vi "Parse Object Content.vi"(8 "error in (no error)":errorcluster, 11 "Response body":string) -> (0 "error out":errorcluster, 3 "Object content":T1[](array[typedef]))   [LabVIEW 2015, in "NI_AWS_S3.lvlib" / "Object.lvclass"]
doc: "Parse out the Contents part of the Response body of a List bucket request."
uses:
  Object.lvclass
  Object Content.ctl
  Storage Class.ctl
  Owner.ctl
  NI_AWS_S3.lvlib
  XML Parsing/NI_XML Parsing.lvlib
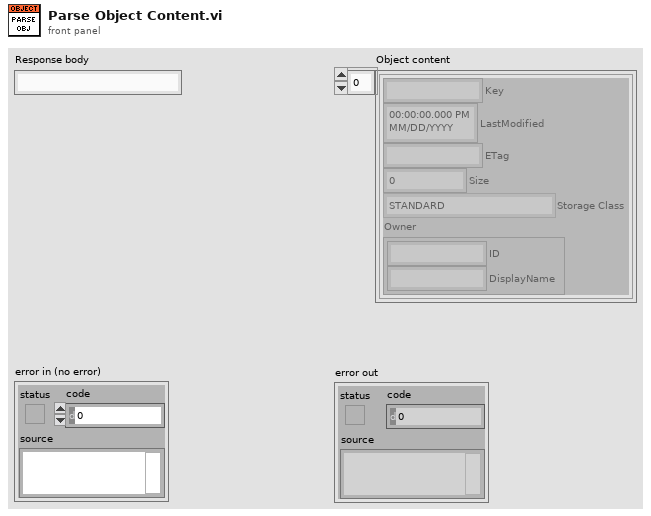
[diagram p1: front panel]
types:
  T1 = typedef "NI_AWS_S3.lvlib/Object Content.ctl" = cluster{"Key":string, "LastModified":timestamp, "ETag":string, "Size":u64, "Storage Class":T2, "Owner":T3}
  T2 = typedef "NI_AWS_S3.lvlib/Storage Class.ctl" = enum16{"STANDARD", "REDUCED_REDUNDANCY"}
  T3 = typedef "NI_AWS_S3.lvlib/Owner.ctl" = cluster{"ID":string, "DisplayName":string}
  T4 = cluster{"[0]":string, "[1]":string, "[2]":string, "[3]":string, "[4]":string}
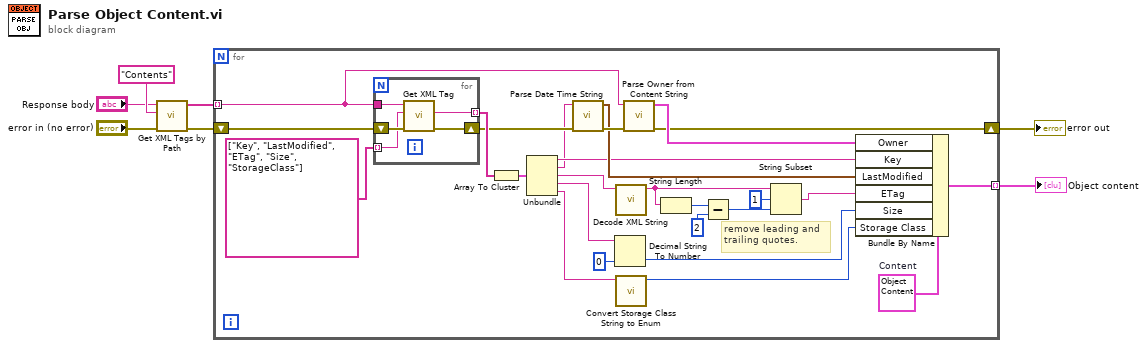
[diagram p0: block diagram]
diagram:
  n1 = call "Get XML Tags by Path.vi"("error in (no error)"="error in (no error)", "Tag path"="Contents", "XML String in"="Response body") -> ("error out"=w5:errorcluster, "Matching tag values"=w6:string[])  [unwired: 7 in]
  n2 = for {
    tunnel: w6 -> [w31] mode=indexing
    shift-right: [w26] -> w2
    shift-left: w5 -> [w33]
    tunnel: [w15] -> w1 mode=indexing
    w28 = T1 {"Key"="", "LastModified"=timestamp(0 s since 1904-01-01), "ETag"="", "Size"=0, "Storage Class"=enum."STANDARD", "Owner"={"ID"="", "DisplayName"=""}}  # Content
    # "remove leading and\ntrailing quotes."
    n3 = for {
      tunnel: string[] ["Key", "LastModified", "ETag", "Size", "StorageClass"] -> [w37] mode=indexing
      tunnel: w31 -> [w36]
      tunnel: [w35] -> w30 mode=indexing
      shift-right: [w34] -> w25
      shift-left: w33 -> [w38]
      n4 = call "Get XML Tag.vi"("error in (no error)"=w38, "Tag name"=w37, "XML String in"=w36) -> ("error out"=w34:errorcluster, "Tag value"=w35:string)  [unwired: 4 in, 3 out]
    }
    n5 = Array To Cluster(array=w30) -> (cluster=w29:T4)
    n6 = Unbundle(w29) -> ("[0]"=w22:string, "[1]"=w21:string, "[2]"=w14:string, "[3]"=w19:string, "[4]"=w17:string)
    n7 = call "Parse Date Time String.vi"("error in (no error)"=w25, "DateTime String"=w21) -> ("error out"=w24:errorcluster, "Time Stamp"=w23:timestamp)  [unwired: 8 in]
    n8 = Decimal String To Number(string=w19, default (0L)=u64 0 ("default (0 I32)")) -> (number=w18:u64)  [unwired: 1 in, 1 out]
    n9 = call "Decode XML String.vi"("String in"=w14) -> ("String out"=w11:string)  [unwired: 10 in]
    n10 = call "Convert Storage Class String to Enum.vi"("Storage Class String"=w17) -> ("Storage Class"=w16:T2)  [unwired: 10 in]
    n11 = call "Parse Owner from Content String.vi"("error in (no error)"=w24, "Content string"=w31) -> ("error out"=w26:errorcluster, "Owner"=w27:T3)  [unwired: 8 in]
    n12 = String Length(string=w11) -> (length=w13:i32)
    n13 = Subtract(x=w13, y=2) -> (x-y=w10:i32)
    n14 = String Subset(string=w11, offset (0)=1, length (rest)=w10) -> (substring=w9:string)
    n15 = Bundle By Name(cluster=w28, "Owner"=w27, "Key"=w22, "LastModified"=w23, "ETag"=w9, "Size"=w18, "Storage Class"=w16) -> (w15:T1)
  }
  "Object content" <- w1
  "error out" <- w2
